vi "ep_Split Vectors Symetrical Components.vi"(8 "error in (no error)":errorcluster, 10 "line voltage? (F)":bool, 11 "one period fundamental vectors":T3(array[cluster])) -> (0 "error out":errorcluster, 3 "spectra symetrical components":T1)   [LabVIEW 2014, in "NI_EP_Power Quality.lvlib"]
uses:
  <vilib>/addons/Electrical Power/PQ/NI_EP_Power Quality.lvlib
  <vilib>/addons/Electrical Power/PQ/Common/Controls/ep_AI Data Channel.ctl
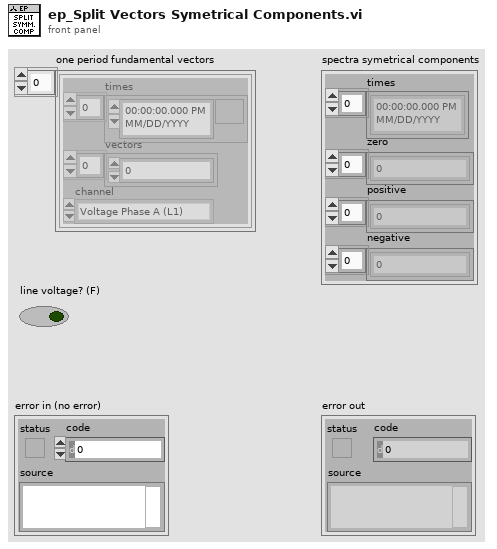
[diagram p1: front panel]
types:
  T1 = cluster{"times":timestamp[], "zero":cdb[], "positive":cdb[], "negative":cdb[]}
  T2 = typedef "NI_EP_Power Quality.lvlib/ep_AI Data Channel.ctl" = enum16{"Voltage Phase A (L1)", "Voltage Phase B (L2)", "Voltage Phase C (L3)", "Voltage Phase N (Neutral)", "Current Phase A (L1)", "Current Phase B (L2)", "Current Phase C (L3)", "Current Phase N (Neutral)"}
  T3 = cluster{"times":timestamp[], "vectors":cdb[], "channel":T2}[]
  T4 = cluster{"times":timestamp[], "vectors":cdb[], "channel":T2}
  T5 = cluster{"times":timestamp[], cdb[], cdb[], cdb[]}
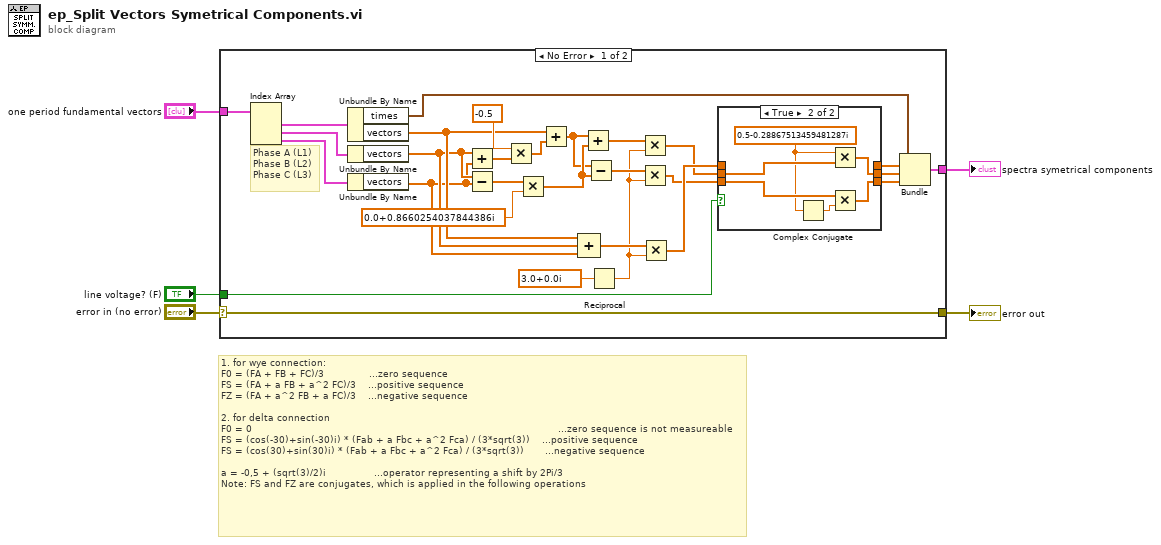
[diagram p0: block diagram]
diagram:
  # "1. for wye connection:\nF0 = (FA + FB + FC)/3               ...zero sequence\nFS = (FA + a FB + a^2 FC)/3    ...positive sequence\nFZ = (FA + a^2 FB + a FC)/3    ...negative sequence\n\n2. for delta connection\nF0 = 0                                                                                                      ...zero sequence is not measureable\nFS = (cos(-30)+sin(-30)i) * (Fab + a Fbc + a^2 Fca) / (3*sqrt(3))    ...positive sequence\nFS = (cos(30)+sin(30)i) * (Fab + a Fbc + a^2 Fca) / (3*sqrt(3))       ...negative sequence\n\na = -0,5 + (sqrt(3)/2)i                ...operator representing a shift by 2Pi/3\nNote: FS and FZ are conjugates, which is applied in the following operations"
  n1 = case shown="No Error" "error in (no error)" {
    selector: "error in (no error)" -> [w13 w44]
    tunnel: "one period fundamental vectors" -> [w30 _]
    tunnel: [w14 _] -> w4
    tunnel: [w13 w44] -> w2
    tunnel: "line voltage? (F)" -> [w6 _]
    frame No Error {
      # "Phase A (L1)\nPhase B (L2)\nPhase C (L3)"
      n2 = Index Array(array=w30) -> (element #1=w32:T4, element #2=w33:T4, element #3=w34:T4)  [unwired: 3 in]
      n3 = Unbundle By Name(w32) -> ("times"=w31:timestamp[], "vectors"=w21:cdb[])
      n4 = Unbundle By Name(w33) -> ("vectors"=w20:cdb[])
      n5 = Unbundle By Name(w34) -> ("vectors"=w19:cdb[])
      n6 = Add(x=w20, y=w19) -> (x+y=w23:cdb[])
      n7 = Subtract(x=w20, y=w19) -> (x-y=w26:cdb[])
      n8 = Multiply(x=-0.5 ("y"), y=w23) -> (x*y=w25:cdb[])
      n9 = Multiply(x=w26, y=cdb 0.0+0.8660254037844386i) -> (x*y=w29:cdb[])
      n10 = Add(x=w21, y=w25) -> (x+y=w28:cdb[])
      n11 = Compound Arithmetic op=ADD(w21, w20, w19) -> (w16:cdb[])
      n12 = Add(x=w28, y=w29) -> (x+y=w18:cdb[])
      n13 = Subtract(x=w28, y=w29) -> (x-y=w17:cdb[])
      n14 = Reciprocal(x=cdb 3.0+0.0i ("y")) -> (1/x=w15:cdb)
      n15 = Multiply(x=w18, y=w15) -> (x*y=w11:cdb[])
      n16 = Multiply(x=w17, y=w15) -> (x*y=w10:cdb[])
      n17 = Multiply(x=w16, y=w15) -> (x*y=w12:cdb[])
      n18 = case shown="True" w6 {
        tunnel: w12 -> [w37 _]
        tunnel: [w37 _] -> w9
        tunnel: w11 -> [w36 w43]
        tunnel: [w36 w42] -> w8
        tunnel: [w35 w40] -> w7
        tunnel: w10 -> [w35 w41]
        frame False {
        }
        frame True {
          w38 = cdb 0.5-0.28867513459481287i
          n19 = Complex Conjugate(1:w38) -> (0:w39:cdb)
          n20 = Multiply(x=w38, y=w43) -> (x*y=w42:cdb[])
          n21 = Multiply(x=w41, y=w39) -> (x*y=w40:cdb[])
        }
      }
      n22 = Bundle("times"=w31, w9, w8, w7) -> (w14:T5)  [unwired: 1 in]
    }
    frame Error {
    }
  }
  "spectra symetrical components" <- w4
  "error out" <- w2
